vi "load_chunk_data.vi"(8 "error in":errorcluster, 9 "Chunk":cluster{T1[]} {"?"."Timestamp" format="%<%.3X>T"}, 10 "File path":path) -> (0 "error out":errorcluster, 2 "Output data":sgl[][][](array[numeric]))   [LabVIEW 2011]
uses:
  ltrace_index.ctl
panel:
  # "Read in trace data for a chunk, returning it directly, and also storing it as though it was a new trace for select_waveforms.vi, etc."
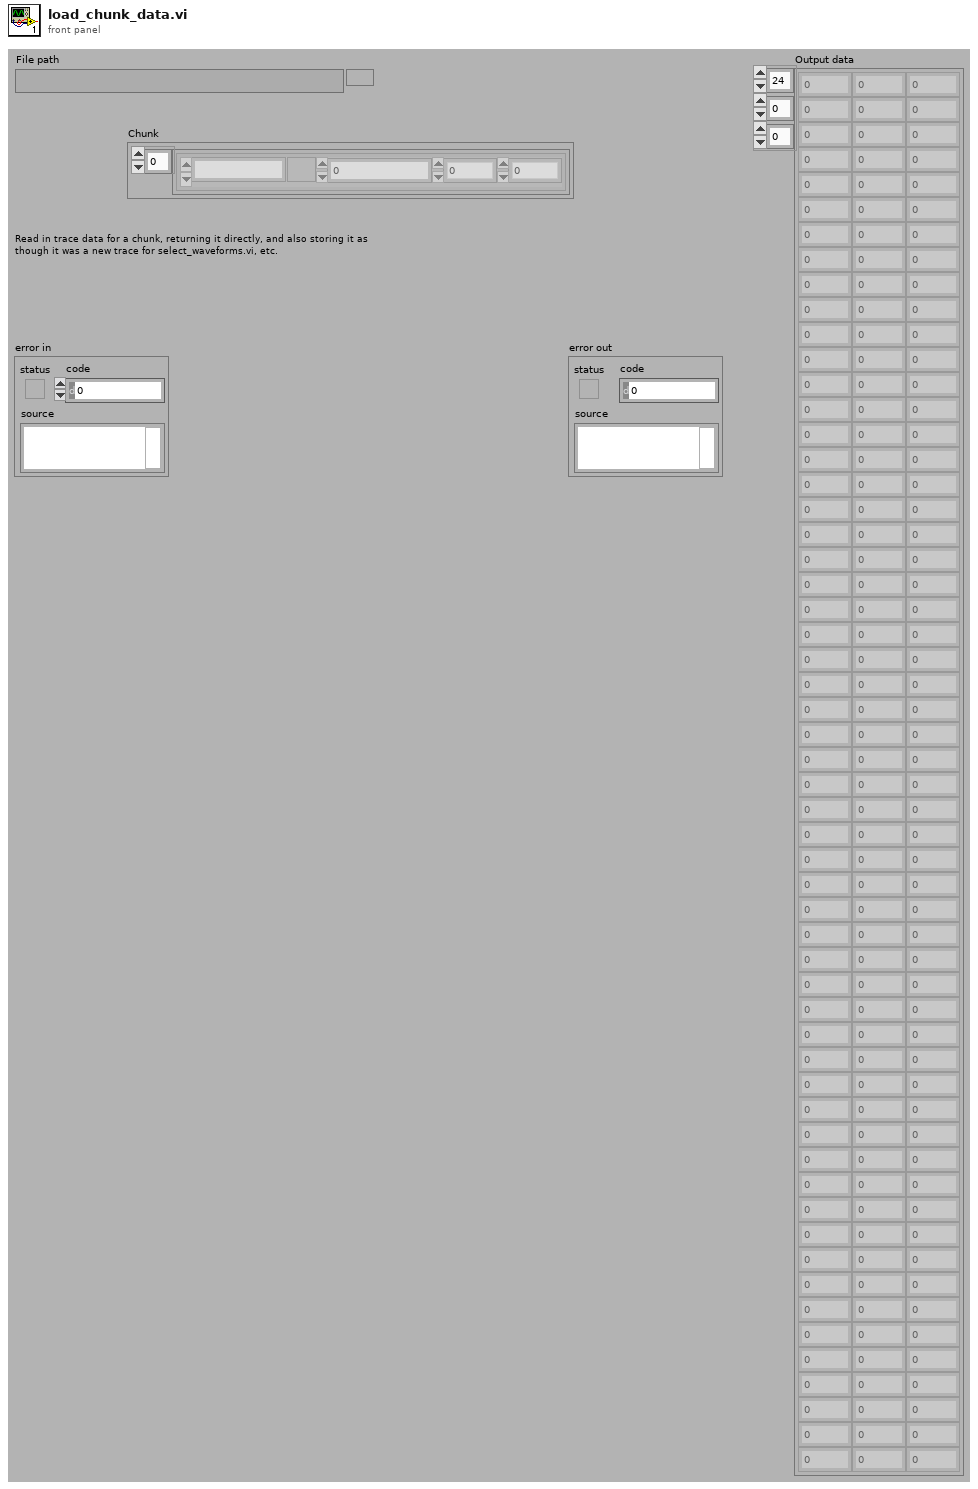
[diagram p1: front panel]
types:
  T1 = typedef "ltrace_index.ctl" = cluster{"Timestamp":timestamp, "Offset":i64, "Sequence":u32, "Flags":u32}
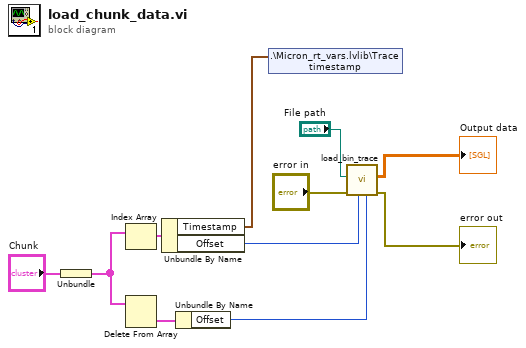
[diagram p0: block diagram]
diagram:
  n1 = Unbundle("Chunk") -> (w10:T1[])
  n2 = Index Array(array=w10) -> (element=w8:T1)  [unwired: 1 in]
  n3 = Delete From Array(array=w10) -> (deleted portion=w9:T1)  [unwired: 2 in, 1 out]
  n4 = Unbundle By Name(w8) -> ("Timestamp"=w1:timestamp, "Offset"=w7:i64)
  n5 = Unbundle By Name(w9) -> ("Offset"=w6:i64)
  n6 = shared-variable ".\\Micron_rt_vars.lvlib\\Trace timestamp"(w1) -> ()  [unwired: 1 in, 1 out]
  n7 = call "load_bin_trace.vi"("Last offset"=w6, "Start offset"=w7, "error in"="error in", "File path"="File path") -> ("error out"=→"error out":errorcluster, "Output data"=→"Output data":sgl[][][])  [unwired: 6 in]
